vi "PH_BackreflectionMeas.panel.vi"(0 "object ref":refnum<vi>, 5 "error in (no error)":errorcluster) -> (19 "error out":errorcluster)   [LabVIEW 2014, in "PH_BackreflectionMeas.lvlib"]
doc: "This a GUI.\n\nLicense Agreement for this software:\n\nCopyright (C)\nGesellschaft für Schwerionenforschung, GSI\nPlanckstr. 1\n64291 Darmstadt\nGermany\n\nContact: D.Beck@gsi.de \n\nThis program is free software; you can redistribute it and/or modify it under the terms of the GNU General Public License as published by the Free Software Foundation; either version 2 of the license, or (at your option) any later version.\n\nThis program is distributed in the hope that it will be useful, but WITHOUT ANYW ARRANTY; without even the implied warranty of MERCHANTABILITY or FITNESS FOR A PARTICULAR PURPOSE. See the GNU General License for more details (http://www.gnu.org).\n\nGesellschaft für Schwerionenforschung, GSI\nPlanckstr. 1, 64291 Darmstadt, Germany\nFor all questions and ideas contact: M.Richter@gsi.de, H.Brand@gsi.de or D.Beck@gsi.de.\nLast update: 18-DEC-2002"
uses:
  PH_BackreflectionMeas.lvlib
  PH_StatusHandler/PH_StatusHandler.GUI element.ctl
  PH_TKTDS-30xx/PH_TKTDS-30xx.Acquisition Config.ctl
  PH_TKTDS-30xx/PH_TKTDS-30xx.Trigger Config.ctl
  PH_TKTDS-30xx/PH_TKTDS-30xx.Channel Config.ctl
  PH_TKTDS-30xx/PH_TKTDS-30xx.GUI Refs.ctl
  CSCore/CSObj/CSObj.lvlib
  PH_Common/PH_Common.lvlib
  CSCore/CSSystem/CSSystemLib/CSSystemLib.lvlib
  PH_TKTDS-30xx/PH_TKTDS-30xx.lvlib
  PH_Class/PH_Class.lvlib
  PH_StatusHandler/PH_StatusHandler.lvlib
panel:
  in  "Save Data":bool
  in  "Get Data":bool
  out "VISA Resource":string
  out "State":u32(colorbox)
  out "PSDB Status":u32(colorbox)=6618880 caption="PSDB"
  in  "Tab Control":T1(tab)
  out "MIRA State":u32(colorbox) caption="BR State"
  in  "Reset warning":bool
  out "High Energy Graph":waveform(dbl)[](graph)
  out "Low Energy Graph":waveform(dbl)[](graph)
  in  "High Energy Channel":T2={"Channel Name"="CH1", "Input Impedance"="MEG", "Max Input Frequency"="TWENTY", "Vertical Coupling"=1, "Channel Enabled"=TRUE, "Probe Attenuation"=1.0, "Vertical Range"=100.0, "Vertical Offset"=0.0} {"Vertical Offset" format="%#_6p"; "Vertical Range" items=["1mV"=0.001, "2mV"=0.002, "5mV"=0.005, "10mV"=0.01, "20mV"=0.02, "50mV"=0.05, "100mV"=0.1, "200mV"=0.2, "500mV"=0.5, "1V"=1.0]; "Probe Attenuation" format="%#.2f"}
  in  "Low Energy Channel":T2={"Channel Name"="CH1", "Input Impedance"="MEG", "Max Input Frequency"="TWENTY", "Vertical Coupling"=1, "Channel Enabled"=TRUE, "Probe Attenuation"=1.0, "Vertical Range"=100.0, "Vertical Offset"=0.0} {"Vertical Offset" format="%#_6p"; "Vertical Range" items=["1mV"=0.001, "2mV"=0.002, "5mV"=0.005, "10mV"=0.01, "20mV"=0.02, "50mV"=0.05, "100mV"=0.1, "200mV"=0.2, "500mV"=0.5, "1V"=1.0]; "Probe Attenuation" format="%#.2f"}
  in  "Trigger":T3={"Source"="CH1", "Slope"=0, "Level [V]"=0.0} {"Level [V]" format="%#_6p"}
  in  "Acquisition Configuration":T4={"Time base"=2e-07, "Record Length"=10000, "Start Time"=0.0, "Type"=0, "Continuous"=FALSE} {"Start Time" format="%#_12p"; "Record Length" items=["500"=500, "10000"=10000]; "Time base" items=["2ns"=2e-09, "4ns"=4e-09, "10ns"=1e-08, "20ns"=2e-08, "40ns"=4e-08, "100ns"=1e-07, "200ns"=2e-07, "400ns"=4e-07, "1µs"=1e-06, "2µs"=2e-06, "4µs"=4e-06, "10µs"=1e-05, "20µs"=2e-05, "40µs"=4e-05, "100µs"=0.0001, "200µs"=0.0002, "400µs"=0.0004, "1ms"=0.001, "2ms"=0.002, "10ms"=0.01, "20ms"=0.02, "40ms"=0.04, "100ms"=0.1, "200ms"=0.2, "400ms"=0.4, "1s"=1.0, "2s"=2.0, "4s"=4.0, "10s"=10.0]}
  in  "Display Intensity":u8=1 min=1 max=100 step=1
  in  "Channel to be positioned":string(combo)="CH1"
  in  "Position":dbl
  out "Status":T5 caption="Enabling State"
  in  "Delete":bool
  in  "Exit":bool
  # "PCS"
  # "3.40"
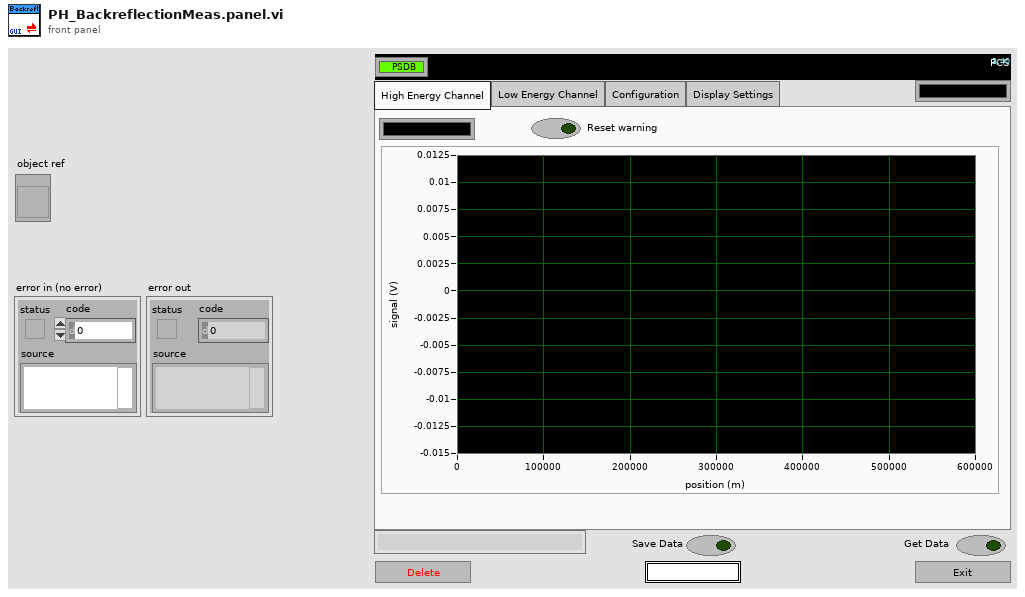
[diagram p1: front panel]
types:
  T1 = enum32{"High Energy Channel", "Low Energy Channel", "Configuration", "Display Settings"}
  T2 = typedef "PH_TKTDS-30xx.lvlib/PH_TKTDS-30xx.Channel Config.ctl" = cluster{"Channel Name":string, "Input Impedance":string, "Max Input Frequency":string, "Vertical Coupling":i32, "Channel Enabled":bool, "Probe Attenuation":dbl, "Vertical Range":dbl, "Vertical Offset":dbl}
  T3 = typedef "PH_TKTDS-30xx.lvlib/PH_TKTDS-30xx.Trigger Config.ctl" = cluster{"Source":string, "Slope":i32, "Level [V]":dbl}
  T4 = typedef "PH_TKTDS-30xx.lvlib/PH_TKTDS-30xx.Acquisition Config.ctl" = cluster{"Time base":dbl, "Record Length":u16, "Start Time":dbl, "Type":i32, "Continuous":bool}
  T5 = typedef "PH_StatusHandler.lvlib/PH_StatusHandler.GUI element.ctl" = u16
  T6 = typedef "PH_TKTDS-30xx.lvlib/PH_TKTDS-30xx.GUI Refs.ctl" = cluster{"Trigger":refnum<vi>, "Acquisition":refnum<vi>, "Graph":refnum<vi>, "State":refnum<vi>, "Delete":refnum<vi>, "Channel to be positioned":refnum<vi>, "Postion":refnum<vi>, "Display Intensity":refnum<vi>, "VISA Resource":refnum<vi>}
  T7 = cluster{"TEK 30xx GUI Refs":T6, "TEK 30xx Channel Refs":refnum<vi>[], "Ref PSDB Status":refnum<vi>}
  T8 = typedef "PH_BackreflectionMeas.lvlib/PH_BackreflectionMeas.i attribute.ctl" = cluster{"GUI Refs":cluster{"Get Data":refnum<vi>, "BR State":refnum<vi>, "Reset warning":refnum<vi>, "Low Energy Graph":refnum<vi>}, "Status":cluster{"Reset Warning":bool}, "Default Low Energy Chan Settings":T2, "Default High Energy Chan Settings":T2, "Default Trigger Settings":T3, "Default Acqu Settings":T4, "Limit [V]":dbl}
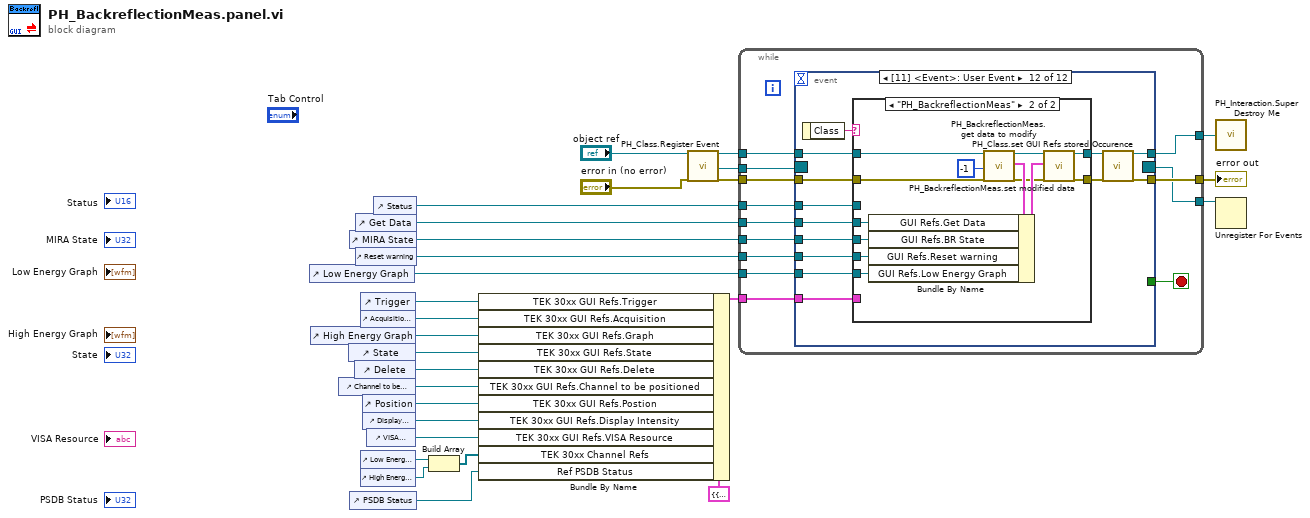
[diagram p0: block diagram]
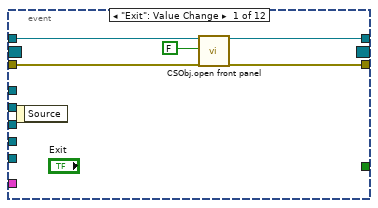
[diagram p2: hidden frame]
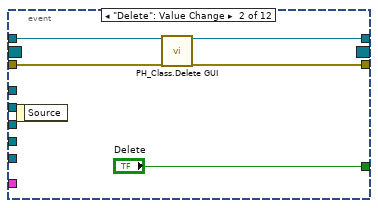
[diagram p3: hidden frame]
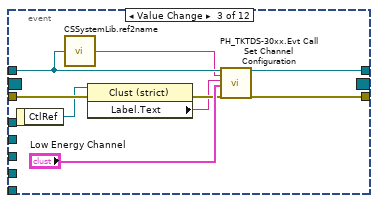
[diagram p4: hidden frame]
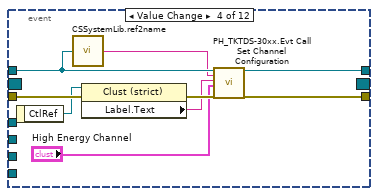
[diagram p5: hidden frame]
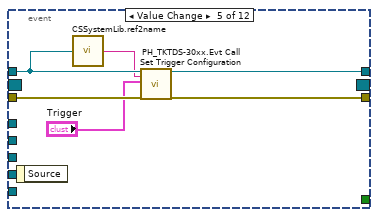
[diagram p6: hidden frame]
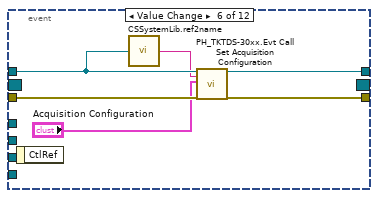
[diagram p7: hidden frame]
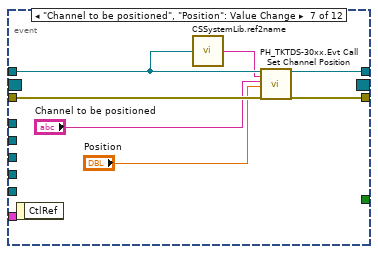
[diagram p8: hidden frame]
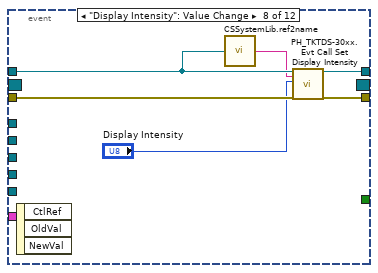
[diagram p9: hidden frame]
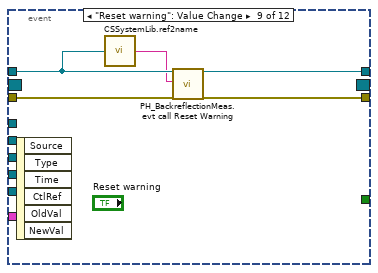
[diagram p10: hidden frame]
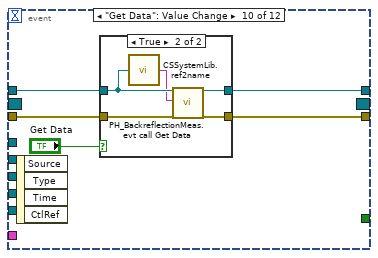
[diagram p11: hidden frame]
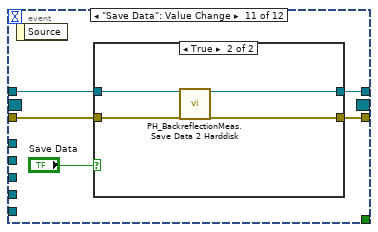
[diagram p13: hidden frame]
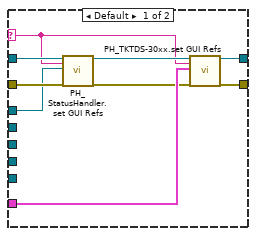
[diagram p15: hidden frame]
diagram:
  n1 = control-ref of="Low Energy Graph"() -> (w5:refnum<vi>)
  n2 = control-ref of="High Energy Graph"() -> (w16:refnum<vi>)
  n3 = control-ref of="Channel to be positioned"() -> (w18:refnum<vi>)
  n4 = control-ref of="State"() -> (w25:refnum<vi>)
  n5 = control-ref of="MIRA State"() -> (w7:refnum<vi>)
  n6 = control-ref of="PSDB Status"() -> (w9:refnum<vi>)
  n7 = control-ref of="Delete"() -> (w26:refnum<vi>)
  n8 = control-ref of="Get Data"() -> (w8:refnum<vi>)
  n9 = control-ref of="Reset warning"() -> (w6:refnum<vi>)
  n10 = control-ref of="Trigger"() -> (w23:refnum<vi>)
  n11 = control-ref of="Acquisition Configuration"() -> (w24:refnum<vi>)
  n12 = control-ref of="Low Energy Channel"() -> (w21:refnum<vi>)
  n13 = control-ref of="High Energy Channel"() -> (w22:refnum<vi>)
  n14 = control-ref of="Position"() -> (w19:refnum<vi>)
  n15 = control-ref of="Display Intensity"() -> (w20:refnum<vi>)
  n16 = control-ref of="VISA Resource"() -> (w17:refnum<vi>)
  n17 = control-ref of="Status"() -> (w1:refnum<vi>)
  n18 = Build Array(w21, w22) -> (w10:refnum<vi>[])
  n19 = Bundle By Name(cluster=T7 {"TEK 30xx GUI Refs"={"Trigger"=refnum, "Acquisition"=refnum, "Graph"=refnum, "State"=refnum, "Delete"=refnum, "Channel to be positioned"=refnum, "Postion"=refnum, "Display Intensity"=refnum, "VISA Resource"=refnum}, "TEK 30xx Channel Refs"=[], "Ref PSDB Status"=refnum} ("GUI Refs"), "TEK 30xx GUI Refs.Trigger"=w23, "TEK 30xx GUI Refs.Acquisition"=w24, "TEK 30xx GUI Refs.Graph"=w16, "TEK 30xx GUI Refs.State"=w25, "TEK 30xx GUI Refs.Delete"=w26, "TEK 30xx GUI Refs.Channel to be positioned"=w18, "TEK 30xx GUI Refs.Postion"=w19, "TEK 30xx GUI Refs.Display Intensity"=w20, "TEK 30xx GUI Refs.VISA Resource"=w17, "TEK 30xx Channel Refs"=w10, "Ref PSDB Status"=w9) -> (w4:T7)
  n20 = call "PH_Class.Register Event.vi"("i ref in"="object ref", "error in (no error)"="error in (no error)") -> ("i ref out"=w15:refnum<vi>, "Event Registration Refnum"=w13:refnum<event-registration>, "error out"=w14:errorcluster)  [unwired: 15 in]
  n21 = while {
    tunnel: w15 -> [w38]
    tunnel: [w37] -> w28
    tunnel: w14 -> [w40]
    tunnel: [w39] -> w27
    tunnel: w13 -> [w36]
    tunnel: [w35] -> w12
    tunnel: w1 -> [w34]
    tunnel: w8 -> [w33]
    tunnel: w7 -> [w32]
    tunnel: w6 -> [w31]
    tunnel: w5 -> [w30]
    tunnel: w4 -> [w29]
    stop <- w41 stop-if-true
    n22 = event shown="[11] <Event>: User Event" {
      selector: w36 -> [_ _ _ _ _ _ _ _ _ _ _ _]
      dyn-events: [_ _ _ _ _ _ _ _ _ _ _ _] -> w35
      timeout: _ -> [_ _ _ _ _ _ _ _ _ _ _ _]
      tunnel: [_ "Delete" _ _ _ _ _ _ _ _ _ _] -> w41
      tunnel: w38 -> [w43 w48 w57 w66 w72 w78 w85 w91 w96 w101 w116 w133]
      tunnel: w40 -> [w46 w50 w60 w69 w75 w81 w88 w94 w99 w104 w115 w132]
      tunnel: [w45 w49 w58 w67 w73 w79 w86 w92 w97 w102 w113 w134] -> w39
      tunnel: [w42 w47 w59 w68 w74 w80 w87 w93 w98 w103 w114 w135] -> w37
      tunnel: w34 -> [_ _ _ _ _ _ _ _ _ _ _ w129]
      tunnel: w33 -> [_ _ _ _ _ _ _ _ _ _ _ w128]
      tunnel: w32 -> [_ _ _ _ _ _ _ _ _ _ _ w127]
      tunnel: w31 -> [_ _ _ _ _ _ _ _ _ _ _ w126]
      tunnel: w30 -> [_ _ _ _ _ _ _ _ _ _ _ w125]
      tunnel: w29 -> [_ _ _ _ _ _ _ _ _ _ _ w123]
      event "Exit": Value Change {
        n23 = event-data() -> ()  [unwired: 1 in, 1 out]
        n24 = call "CSObj.open front panel.vi"("i ref in"=w43, "frontPanelOpen"=FALSE ("front panel open"), "error in (no error)"=w46) -> ("i ref out"=w42:refnum<vi>, "error out"=w45:errorcluster)  [unwired: 15 in]
      }
      event "Delete": Value Change {
        n25 = event-data() -> ()  [unwired: 1 in, 1 out]
        n26 = call "PH_Class.Delete GUI.vi"("VI in"=w48, "error in (no error)"=w50) -> ("VI out"=w47:refnum<vi>, "error out"=w49:errorcluster)  [unwired: 16 in]
      }
      event Value Change {
        n27 = event-data() -> ("CtlRef"=w53:refnum<vi>)  [unwired: 1 in]
        n28 = call "CSSystemLib.ref2name.vi"("obj refnum"=w57) -> ("name"=w56:string)
        n29 = property class="Clust (strict)"(reference=w53, error in=w60) -> (error out=w54:errorcluster, "Label.Text"=w52:string)  [unwired: 1 out]
        n30 = call "PH_TKTDS-30xx.Evt Call Set Channel Configuration.vi"("i ref in"=w57, "Instance"=w56, "GUI Element Name"=w52, "Channel Configuration"="Low Energy Channel", "error in (no error)"=w54) -> ("i ref out"=w59:refnum<vi>, "error out"=w58:errorcluster)  [unwired: 13 in]
      }
      event Value Change {
        n31 = event-data() -> ("CtlRef"=w63:refnum<vi>)  [unwired: 1 in]
        n32 = call "CSSystemLib.ref2name.vi"("obj refnum"=w66) -> ("name"=w65:string)
        n33 = property class="Clust (strict)"(reference=w63, error in=w69) -> (error out=w64:errorcluster, "Label.Text"=w61:string)  [unwired: 1 out]
        n34 = call "PH_TKTDS-30xx.Evt Call Set Channel Configuration.vi"("i ref in"=w66, "Instance"=w65, "GUI Element Name"=w61, "Channel Configuration"="High Energy Channel", "error in (no error)"=w64) -> ("i ref out"=w68:refnum<vi>, "error out"=w67:errorcluster)  [unwired: 13 in]
      }
      event Value Change {
        n35 = event-data() -> ()  [unwired: 1 in, 1 out]
        n36 = call "CSSystemLib.ref2name.vi"("obj refnum"=w72) -> ("name"=w71:string)
        n37 = call "PH_TKTDS-30xx.Evt Call Set Trigger Configuration.vi"("i ref in"=w72, "Instance"=w71, "Trigger Configuration"="Trigger", "error in (no error)"=w75) -> ("i ref out"=w74:refnum<vi>, "error out"=w73:errorcluster)  [unwired: 14 in]
      }
      event Value Change {
        n38 = event-data() -> ()  [unwired: 1 in, 1 out]
        n39 = call "CSSystemLib.ref2name.vi"("obj refnum"=w78) -> ("name"=w77:string)
        n40 = call "PH_TKTDS-30xx.Evt Call Set Acquisition Configuration.vi"("i ref in"=w78, "Instance"=w77, "Acquisition Configuration"="Acquisition Configuration", "error in (no error)"=w81) -> ("i ref out"=w80:refnum<vi>, "error out"=w79:errorcluster)  [unwired: 14 in]
      }
      event "Channel to be positioned", "Position": Value Change {
        n41 = event-data() -> ()  [unwired: 1 in, 1 out]
        n42 = call "CSSystemLib.ref2name.vi"("obj refnum"=w85) -> ("name"=w84:string)
        n43 = call "PH_TKTDS-30xx.Evt Call Set Channel Position.vi"("i ref in"=w85, "Instance"=w84, "Channel to be positioned"="Channel to be positioned", "Position"="Position", "error in (no error)"=w88) -> ("i ref out"=w87:refnum<vi>, "error out"=w86:errorcluster)  [unwired: 13 in]
      }
      event "Display Intensity": Value Change {
        n44 = event-data() -> ()  [unwired: 1 in, 3 out]
        n45 = call "CSSystemLib.ref2name.vi"("obj refnum"=w91) -> ("name"=w90:string)
        n46 = call "PH_TKTDS-30xx.Evt Call Set Display Intensity.vi"("i ref in"=w91, "Instance"=w90, "Display Intensity"="Display Intensity", "error in (no error)"=w94) -> ("i ref out"=w93:refnum<vi>, "error out"=w92:errorcluster)  [unwired: 14 in]
      }
      event "Reset warning": Value Change {
        n47 = event-data() -> ()  [unwired: 1 in, 6 out]
        n48 = call "CSSystemLib.ref2name.vi"("obj refnum"=w96) -> ("name"=w95:string)
        n49 = call "PH_BackreflectionMeas.evt call Reset Warning.vi"("i ref in"=w96, "Instance"=w95, "error in (no error)"=w99) -> ("i ref out"=w98:refnum<vi>, "error out"=w97:errorcluster)  [unwired: 15 in]
      }
      event "Get Data": Value Change {
        n50 = event-data() -> ()  [unwired: 1 in, 4 out]
        n51 = case shown="True" "Get Data" {
          tunnel: w104 -> [w105 w111]
          tunnel: [w106 w110] -> w103
          tunnel: [w105 w109] -> w102
          tunnel: w101 -> [w106 w108]
          frame False {
          }
          frame True {
            n52 = call "CSSystemLib.ref2name.vi"("obj refnum"=w108) -> ("name"=w107:string)
            n53 = call "PH_BackreflectionMeas.evt call Get Data.vi"("i ref in"=w108, "Instance"=w107, "error in (no error)"=w111) -> ("i ref out"=w110:refnum<vi>, "error out"=w109:errorcluster)  [unwired: 15 in]
          }
        }
      }
      event "Save Data": Value Change {
        n54 = event-data() -> ()  [unwired: 1 in, 1 out]
        n55 = case shown="True" "Save Data" {
          tunnel: w116 -> [w118 w120]
          tunnel: w115 -> [w117 w121]
          tunnel: [w118 w119] -> w114
          tunnel: [w117 w122] -> w113
          frame False {
          }
          frame True {
            n56 = call "PH_BackreflectionMeas.Save Data 2 Harddisk.vi"("i ref in"=w120, "error in"=w121) -> ("i ref out"=w119:refnum<vi>, "error out"=w122:errorcluster)  [unwired: 16 in]
          }
        }
      }
      event User Event {
        n57 = event-data() -> ("Class"=w124:string)  [unwired: 1 in]
        n58 = case shown="\"PH_BackreflectionMeas\"" w124 {
          selector: w124 -> [w137 _]
          tunnel: w133 -> [w139 w152]
          tunnel: w132 -> [w143 w151]
          tunnel: [w144 w150] -> w131
          tunnel: [w142 w149] -> w130
          tunnel: w129 -> [w136 _]
          tunnel: w128 -> [_ w148]
          tunnel: w127 -> [_ w147]
          tunnel: w126 -> [_ w146]
          tunnel: w125 -> [_ w145]
          tunnel: w123 -> [w141 _]
          frame Default {
            n59 = call "PH_StatusHandler.set GUI Refs.vi"("i ref in"=w139, "Class"=w137, "GUI Ref"=w136, "error in (no error)"=w143) -> ("i ref out"=w138:refnum<vi>, "error out"=w140:errorcluster)  [unwired: 14 in]
            n60 = call "PH_TKTDS-30xx.set GUI Refs.vi"("i ref in"=w138, "Class"=w137, "GUI Refs"=w141, "error in (no error)"=w140) -> ("i ref out"=w144:refnum<vi>, "error out"=w142:errorcluster)  [unwired: 14 in]
          }
          frame "PH_BackreflectionMeas" {
            n61 = call "PH_BackreflectionMeas.get data to modify.vi"("i ref in"=w152, "ms timeout (10000)"=-1, "error in (no error)"=w151) -> ("i ref out"=w153:refnum<vi>, "i attribute"=w155:T8, "error out"=w154:errorcluster)  [unwired: 13 in, 1 out]
            n62 = Bundle By Name(cluster=w155, "GUI Refs.Get Data"=w148, "GUI Refs.BR State"=w147, "GUI Refs.Reset warning"=w146, "GUI Refs.Low Energy Graph"=w145) -> (w156:T8)
            n63 = call "PH_BackreflectionMeas.set modified data.vi"("i ref in"=w153, "i attribute"=w156, "error in (no error)"=w154) -> ("i ref out"=w150:refnum<vi>, "error out"=w149:errorcluster)  [unwired: 15 in]
          }
        }
        n64 = call "PH_Class.set GUI Refs stored Occurence.vi"("i ref in"=w131, "error in (no error)"=w130) -> ("i ref out"=w135:refnum<vi>, "error out"=w134:errorcluster)  [unwired: 16 in]
      }
    }
  }
  "error out" <- w27
  n65 = call "PH_Interaction.Super Destroy Me.vi"("i ref out"=w28) -> ()
  n66 = Unregister For Events(event registration refnum=w12) -> ()  [unwired: 1 in, 1 out]
